vi "To Value.vi"(8 "error in (no error)":errorcluster, 10 "PV Data in":refnum<class "PV Data.lvclass">, 11 "NT Enum in":refnum<class "NT Enum.lvclass">) -> (0 "error out":errorcluster, 2 "PV Data out":refnum<class "PV Data.lvclass">, 3 "NT Enum out":refnum<class "NT Enum.lvclass">)   [LabVIEW 2020, in "PV Access.lvlib" / "PV Data.lvlib" / "NT Enum.lvclass"]
uses:
  NT Enum.lvclass
  PV Data/PV Data.lvclass
  NT Base/NT Base.lvclass
  NT Enum.lvclass/NT Enum.ctl
  PV Data/Write Field (I32).vi
  PV Data/Write Field (String Array).vi
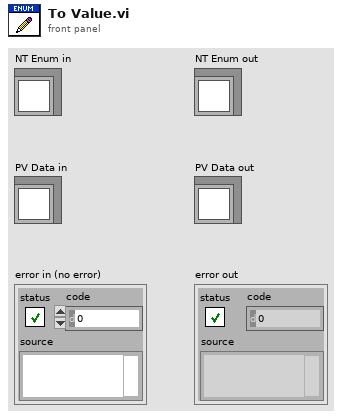
[diagram p1: front panel]
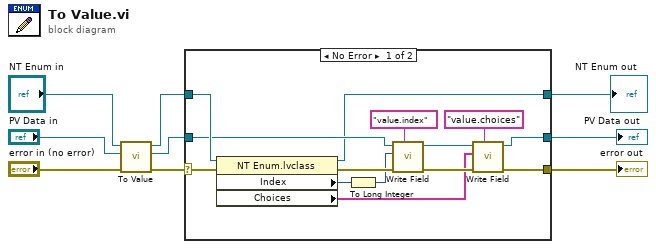
[diagram p0: block diagram]
diagram:
  n1 = call-parent "To Value.vi"("error in (no error)"="error in (no error)", "PV Data in"="PV Data in", "NT Base in"="NT Enum in") -> ("error out"=w3:errorcluster, "PV Data out"=w2:refnum<class "PV Data.lvclass">, "NT Base out"=w1:refnum<class "NT Enum.lvclass">)  [unwired: 6 in]
  n2 = case shown="No Error" w3 {
    selector: w3 -> [w22 w24]
    tunnel: [w17 w24] -> w9
    tunnel: [w13 w25] -> w8
    tunnel: w2 -> [w15 w25]
    tunnel: w1 -> [w23 w26]
    tunnel: [w12 w26] -> w7
    frame No Error {
      n3 = property class="NT Enum.lvclass"(reference=w23, error in=w22) -> (reference out=w12:refnum<class "NT Enum.lvclass">, error out=w21:errorcluster, "Index"=w11:u16, "Choices"=w14:string[])
      n4 = To Long Integer(number=w11) -> (32bit integer=w10:i32)
      n5 = call-poly "Write Field.vi"("field name"="value.index", "error in"=w21, "value"=w10, "PV Data in"=w15) -> ("error out"=w18:errorcluster, "PV Data out"=w16:refnum<class "PV Data.lvclass">)  [unwired: 5 in, 1 out]
      n6 = call-poly "Write Field.vi"("field name"="value.choices", "error in"=w18, "value"=w14, "PV Data in"=w16) -> ("error out"=w17:errorcluster, "PV Data out"=w13:refnum<class "PV Data.lvclass">)  [unwired: 5 in, 1 out]
    }
    frame Error {
    }
  }
  "error out" <- w9
  "NT Enum out" <- w7
  "PV Data out" <- w8
